vi "Page_Advanced_ReadAll.vi"(6 "ctl references":T1, 8 "error in (no error)":errorcluster, 10 "Calculated IncludeHWConfig":bool, 11 "AB_InteropAssembly in":refnum<class "AB_InteropAssembly.lvclass">) -> (0 "error out":errorcluster, 3 "AB_InteropAssembly out":refnum<class "AB_InteropAssembly.lvclass">)   [LabVIEW 2020, in "AB_InteropAssembly.lvclass"]
uses:
  <vilib>/AppBuilder/AB_Classes/InteropAssembly/AB_InteropAssembly.lvclass
  <resource>/Framework/Providers/Builds/AppBuilder/AB_UI_Page_Advanced_References.ctl
  <vilib>/AppBuilder/AB_Classes/InteropAssembly/AB_InteropAssembly.lvclass/AB_InteropAssembly.ctl
  <vilib>/AppBuilder/AB_Classes/Application/AB_Application.lvclass
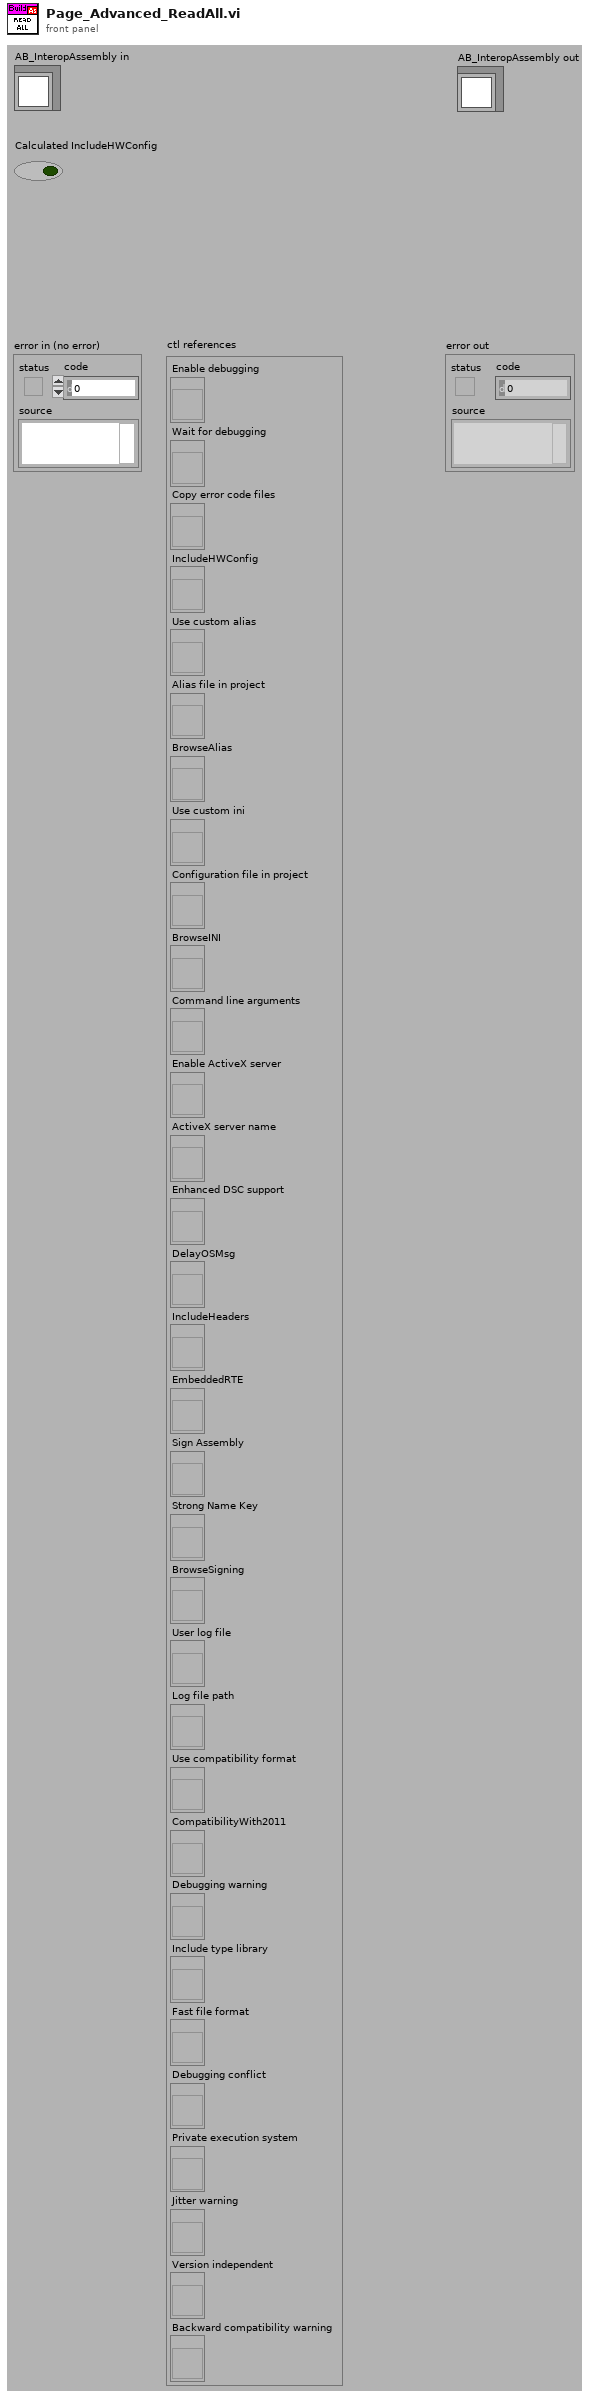
[diagram p1: front panel]
types:
  T1 = typedef "AB_UI_Page_Advanced_References.ctl" = cluster{"Enable debugging":refnum<vi>, "Wait for debugging":refnum<vi>, "Copy error code files":refnum<vi>, "IncludeHWConfig":refnum<vi>, "Use custom alias":refnum<vi>, "Alias file in project":refnum<vi>, "BrowseAlias":refnum<vi>, "Use custom ini":refnum<vi>, "Configuration file in project":refnum<vi>, "BrowseINI":refnum<vi>, "Command line arguments":refnum<vi>, "Enable ActiveX server":refnum<vi>, "ActiveX server name":refnum<vi>, "Enhanced DSC support":refnum<vi>, "DelayOSMsg":refnum<vi>, "IncludeHeaders":refnum<vi>, "EmbeddedRTE":refnum<vi>, "Sign Assembly":refnum<vi>, "Strong Name Key":refnum<vi>, "BrowseSigning":refnum<vi>, "User log file":refnum<vi>, "Log file path":refnum<vi>, "Use compatibility format":refnum<vi>, "CompatibilityWith2011":refnum<vi>, "Debugging warning":refnum<vi>, "Include type library":refnum<vi>, "Fast file format":refnum<vi>, "Debugging conflict":refnum<vi>, "Private execution system":refnum<vi>, "Jitter warning":refnum<vi>, "Version independent":refnum<vi>, "Backward compatibility warning":refnum<vi>}
  T2 = enum8{"Enabled", "Disabled", "Disabled and Grayed Out"}
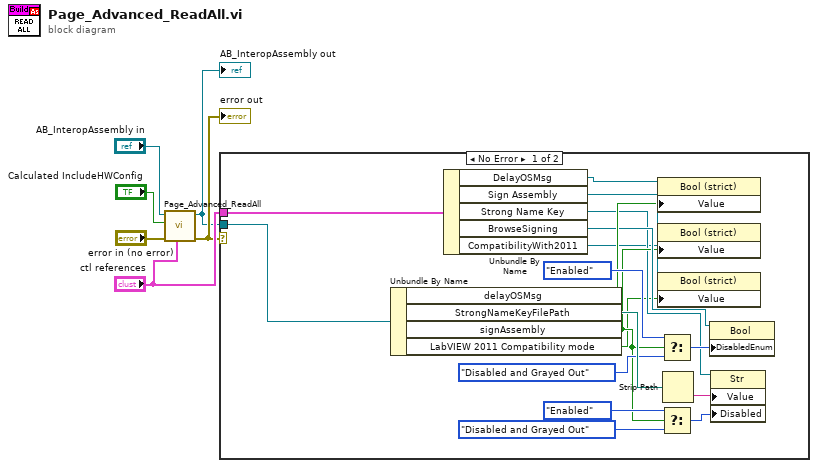
[diagram p0: block diagram]
diagram:
  n1 = call-parent "Page_Advanced_ReadAll.vi"("ctl references"="ctl references", "error in (no error)"="error in (no error)", "Calculated IncludeHWConfig"="Calculated IncludeHWConfig", "AB_Application in"="AB_InteropAssembly in") -> ("error out"=w3:errorcluster, "AB_Application out"=w1:refnum<class "AB_InteropAssembly.lvclass">)  [unwired: 6 out]
  "error out" <- w3
  "AB_InteropAssembly out" <- w1
  n2 = case shown="No Error" w3 {
    tunnel: w1 -> [w24 _]
    tunnel: "ctl references" -> [w23 _]
    frame No Error {
      n3 = Unbundle By Name(w24) -> ("delayOSMsg"=w15:bool, "StrongNameKeyFilePath"=w21:path, "signAssembly"=w12:bool, "LabVIEW 2011 Compatibility mode"=w7:bool)
      n4 = Unbundle By Name(w23) -> ("DelayOSMsg"=w10:refnum<vi>, "Sign Assembly"=w22:refnum<vi>, "Strong Name Key"=w11:refnum<vi>, "BrowseSigning"=w14:refnum<vi>, "CompatibilityWith2011"=w8:refnum<vi>)
      n5 = property class="Bool (strict)"(reference=w10, "Value"=w15) -> ()  [unwired: 1 in, 2 out]
      n6 = property class="Bool (strict)"(reference=w22, "Value"=w12) -> ()  [unwired: 1 in, 2 out]
      n7 = property class="Bool (strict)"(reference=w8, "Value"=w7) -> ()  [unwired: 1 in, 2 out]
      n8 = Select(t=T2."Enabled" ("Disabled"), s=w12, f=T2."Disabled and Grayed Out" ("Disabled")) -> (s? t:f=w13:T2)
      n9 = Select(t=T2."Enabled" ("Disabled"), s=w12, f=T2."Disabled and Grayed Out" ("Disabled")) -> (s? t:f=w9:T2)
      n10 = Strip Path(path=w21) -> (name=w20:string)  [unwired: 1 out]
      n11 = property class="Bool"(reference=w14, "DisabledEnum"=w13) -> ()  [unwired: 1 in, 2 out]
      n12 = property class="Str"(reference=w11, "Value"=w20, "Disabled"=w9) -> ()  [unwired: 1 in, 2 out]
    }
    frame Error {
    }
  }
